vi "Parse Tree Parameters.vi"(8 "error in":errorcluster, 11 "Item Ref in":T4 format="%.0x") -> (0 "error out":errorcluster, 2 "Parameter References":T4[](array[typedef]) format="%.0x", 3 "Item Ref out":T4 format="%.0x", 4 "Parameter Driver Data":T1 {"Num Bits" min=1 max=32; "Start Bit" min=8 max=31})   [LabVIEW 2012, in "AIT 429 Engine.lvlib"]
uses:
  <vilib>/NI Veristand/Custom Device API/Custom Device Item Ref.ctl
  RT Controls/RT Param Setting.ctl
  Shared/Controls and Global/Start Bit.ctl
  Shared/Controls and Global/Number of Bits.ctl
  <vilib>/NI Veristand/Custom Device Tools/Custom Device Utility Library/NI VeriStand - Search for All Items by GUID.vi
  Shared/Controls and Global/Global.vi
  <vilib>/NI Veristand/Custom Device API/Get Item Property (Double).vi
  <vilib>/NI Veristand/Custom Device API/Get Item Property (Boolean).vi
  <vilib>/NI Veristand/Custom Device API/Get Item Property (I32).vi
  AIT 429 Engine.lvlib
  <vilib>/NI Veristand/Custom Device API/Custom Device API.lvlib
  <vilib>/NI Veristand/Custom Device Tools/Custom Device Utility Library/Custom Device Utility Library.lvlib
  ARINC 429 Shared.lvlib
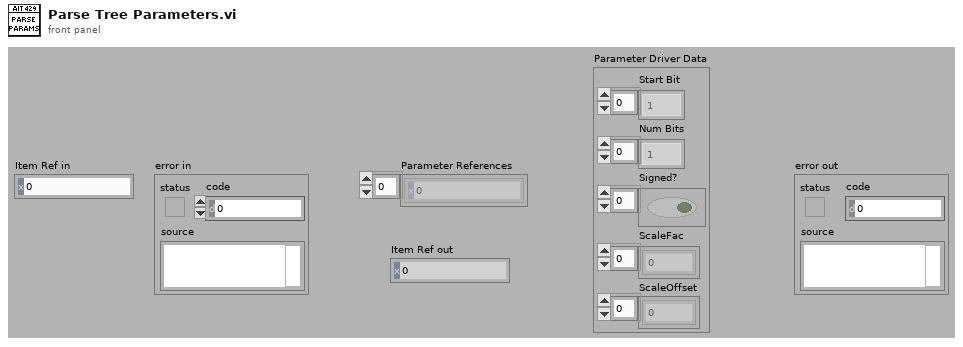
[diagram p1: front panel]
types:
  T1 = typedef "AIT 429 Engine.lvlib/RT Param Setting.ctl" = cluster{"Start Bit":T2[], "Num Bits":T3[], "Signed?":bool[], "ScaleFac":dbl[], "ScaleOffset":dbl[]}
  T2 = typedef "ARINC 429 Shared.lvlib/Start Bit.ctl" = i32
  T3 = typedef "ARINC 429 Shared.lvlib/Number of Bits.ctl" = i32
  T4 = typedef "Custom Device API.lvlib/Custom Device Item Ref.ctl" = u64
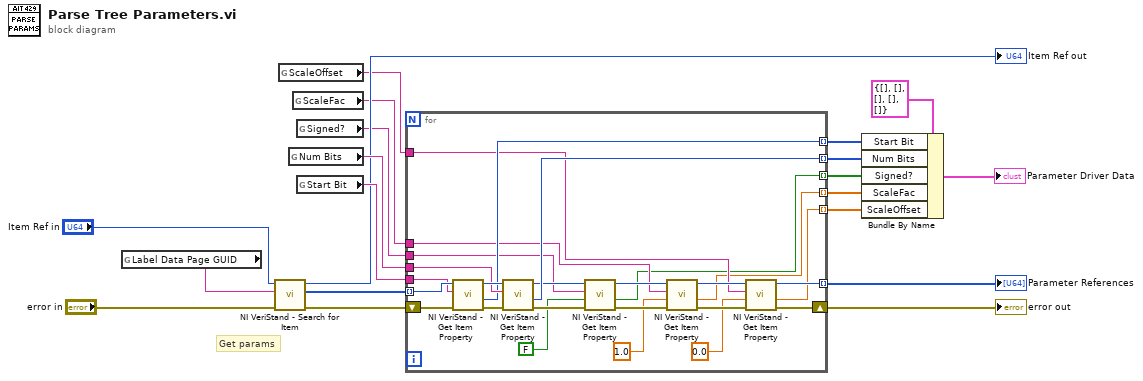
[diagram p0: block diagram]
diagram:
  # "Get params"
  n1 = global read "Global.vi" "Label Data Page GUID"() -> (w18:string)
  n2 = call-poly <vilib>:"NI VeriStand - Search for Item.vi"("error in"="error in", "Item GUID"=w18, "Section Ref in"="Item Ref in") -> ("error out"=w15:errorcluster, "Item Refs"=w14:T4[], "Section Ref out"=→"Item Ref out":T4)  [unwired: 5 in, 1 out]
  n3 = global read "Global.vi" "ScaleOffset"() -> (w6:string)
  n4 = global read "Global.vi" "Num Bits"() -> (w20:string)
  n5 = global read "Global.vi" "ScaleFac"() -> (w7:string)
  n6 = global read "Global.vi" "Signed?"() -> (w8:string)
  n7 = global read "Global.vi" "Start Bit"() -> (w19:string)
  n8 = for {
    shift-right: [w33] -> w13
    shift-left: w15 -> [w45]
    tunnel: w14 -> [w44] mode=indexing
    tunnel: w19 -> [w41]
    tunnel: w20 -> [w40]
    tunnel: [w39] -> w11 mode=indexing
    tunnel: [w38] -> w10 mode=indexing
    tunnel: [w34] -> w9 mode=indexing
    tunnel: w8 -> [w29]
    tunnel: w7 -> [w27]
    tunnel: w6 -> [w25]
    tunnel: [w23] -> w5 mode=indexing
    tunnel: [w22] -> w4 mode=indexing
    tunnel: [w21] -> w3 mode=indexing
    n9 = call-poly <vilib>:"NI VeriStand - Get Item Property.vi"("error in (no error)"=w45, "Property Name"=w41, "Item Ref in"=w44) -> ("error out"=w43:errorcluster, "Value"=w39:i32, "Item Ref out"=w42:T4)  [unwired: 5 in, 1 out]
    n10 = call-poly <vilib>:"NI VeriStand - Get Item Property.vi"("error in (no error)"=w43, "Property Name"=w40, "Item Ref in"=w42) -> ("error out"=w30:errorcluster, "Value"=w38:i32, "Item Ref out"=w37:T4)  [unwired: 5 in, 1 out]
    n11 = call-poly <vilib>:"NI VeriStand - Get Item Property.vi"("error in (no error)"=w30, "Default Value"=FALSE, "Property Name"=w29, "Item Ref in"=w37) -> ("error out"=w31:errorcluster, "Value"=w23:bool, "Item Ref out"=w36:T4)  [unwired: 4 in, 1 out]
    n12 = call-poly <vilib>:"NI VeriStand - Get Item Property.vi"("error in (no error)"=w31, "Default Value"=1.0, "Property Name"=w27, "Item Ref in"=w36) -> ("error out"=w32:errorcluster, "Value"=w22:dbl, "Item Ref out"=w35:T4)  [unwired: 4 in, 1 out]
    n13 = call-poly <vilib>:"NI VeriStand - Get Item Property.vi"("error in (no error)"=w32, "Default Value"=0.0, "Property Name"=w25, "Item Ref in"=w35) -> ("error out"=w33:errorcluster, "Value"=w21:dbl, "Item Ref out"=w34:T4)  [unwired: 4 in, 1 out]
  }
  "error out" <- w13
  "Parameter References" <- w9
  n14 = Bundle By Name(cluster=T1 {"Start Bit"=[], "Num Bits"=[], "Signed?"=[], "ScaleFac"=[], "ScaleOffset"=[]} ("Param Setting"), "Start Bit"=w11, "Num Bits"=w10, "Signed?"=w5, "ScaleFac"=w4, "ScaleOffset"=w3) -> (→"Parameter Driver Data":T1)
